vi "BRig_dataLC_Selection_PreR_Count_l1.vi"() -> (2 "output_Selection_PreR_Count":i32)   [LabVIEW 2014]
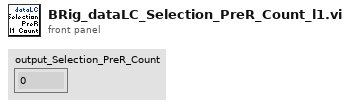
[diagram p1: front panel]
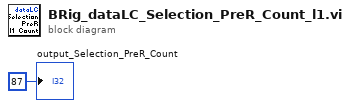
[diagram p0: block diagram]
diagram:
  "output_Selection_PreR_Count" <- 87 ("output_iBlock")
